vi "Interpolated Fluid Properties.vi"(0 "Xi":dbl[](array[numeric]), 5 "Yi":dbl[](array[numeric]), 12 "file path (dialog if empty)":path=path "C:/LabView/CO2 properties from 250 to 400 K and 8 to 15 MPa.txt", 13 "reload?":bool) -> (8 "Zi 1":dbl[](array[numeric]), 10 "Zi 2":dbl[](array[numeric]), 15 "Zi 3":dbl[](array[numeric]))   [LabVIEW 2020]
uses:
  f9a0f065-e32f-4a9d-9d50-07fda239758b.vi
  fc243c30-5152-400b-8647-591f757cc8b1.vi
  5e9bb687-0e7f-4660-b8cc-9489864c6cfa.vi
  <vilib>/Utility/file.llb/Read Delimited Spreadsheet (DBL).vi
  <vilib>/gmath/interp.llb/Interpolate 2D Scattered (1D).vi
  <vilib>/gmath/NI_AAL_Interpolation.lvlib
panel:
  out "Heartbeat":u32(knob) scale=0.0..1000.0 scale format="%#.0f"
  in  "stop":bool
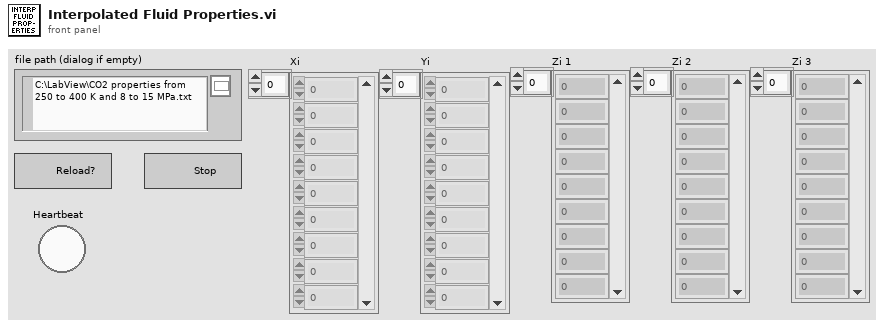
[diagram p1: front panel]
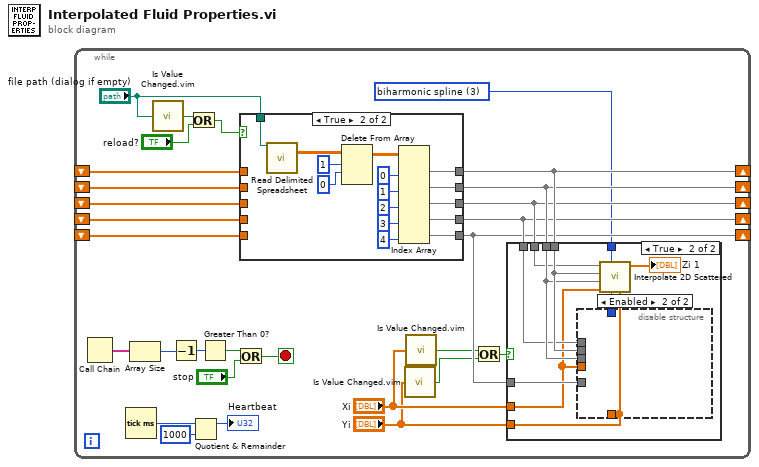
[diagram p0: block diagram]
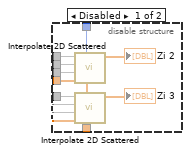
[diagram p3: hidden frame]
diagram:
  n1 = while {
    shift-right: [w25] -> _
    shift-left: _ -> [w20]
    shift-right: [w26] -> _
    shift-left: _ -> [w21]
    shift-right: [w27] -> _
    shift-left: _ -> [w22]
    shift-right: [w29] -> _
    shift-left: _ -> [w24]
    shift-right: [w28] -> _
    shift-left: _ -> [w23]
    stop <- w13 stop-if-true
    w19 = 3 items=["nearest", "linear", "cubic", "biharmonic spline "] ("method")
    n2 = Call Chain() -> (call chain=w14:string[])
    n3 = Tick Count (ms)() -> (millisecond timer value=w8:u32)
    n4 = Array Size(array=w14) -> (size(s)=w15:i32)
    n5 = call "Is Value Changed.vim"("value"="file path (dialog if empty)") -> ("changed or first call?"=w11:bool)
    n6 = Decrement(x=w15) -> (x-1=w16:i32)
    n7 = Or(x=w11, y="reload?") -> (x .or. y?=w10:bool)
    n8 = Quotient & Remainder(x=w8, y=u32 1000) -> (x-y*floor(x/y)=→"Heartbeat":u32)  [unwired: 1 out]
    n9 = Greater Than 0?(x=w16) -> (x > 0?=w17:bool)
    n10 = Or(x=w17, y="stop") -> (x .or. y?=w13:bool)
    n11 = case shown="True" w10 {
      tunnel: [w52 w61] -> w29
      tunnel: [w51 w60] -> w28
      tunnel: [w50 w59] -> w27
      tunnel: [w49 w58] -> w26
      tunnel: [w48 w57] -> w25
      tunnel: w24 -> [w52 _]
      tunnel: w23 -> [w51 _]
      tunnel: w22 -> [w50 _]
      tunnel: w21 -> [w49 _]
      tunnel: w20 -> [w48 _]
      tunnel: "file path (dialog if empty)" -> [_ w56]
      frame False {
      }
      frame True {
        n12 = call-poly <vilib>:"Read Delimited Spreadsheet.vi"("file path (dialog if empty)"=w56) -> ("all rows"=w67:dbl[][])  [unwired: 9 in, 5 out]
        n13 = Delete From Array(array=w67, length=1, index (row)=0) -> (array with subset deleted=w55:dbl[][])  [unwired: 1 in, 1 out]
        n14 = Index Array(array=w55, index (col) #1=0 ("disabled index (col)"), index (col) #2=1 ("index (col)"), index (col) #3=2 ("index (col)"), index (col) #4=3 ("index (col)"), index (col) #5=4 ("index (col)")) -> (element #1=w61:dbl[], element #2=w60:dbl[], element #3=w59:dbl[], element #4=w58:dbl[], element #5=w57:dbl[])  [unwired: 5 in]
      }
    }
    n15 = call "Is Value Changed.vim"("value"="Yi") -> ("changed or first call?"=w1:bool)
    n16 = call "Is Value Changed.vim"("value"="Xi") -> ("changed or first call?"=w2:bool)
    n17 = Or(x=w2, y=w1) -> (x .or. y?=w5:bool)
    n18 = case shown="True" w5 {
      tunnel: w29 -> [_ w38]
      tunnel: w28 -> [_ w37]
      tunnel: w27 -> [_ w36]
      tunnel: w26 -> [_ w35]
      tunnel: w25 -> [_ w34]
      tunnel: "Xi" -> [_ w33]
      tunnel: "Yi" -> [_ w32]
      tunnel: w19 -> [_ w31]
      frame False {
      }
      frame True {
        n19 = disable-structure shown="Enabled" {
          disable-tunnel: w38 -> [w47 _]
          disable-tunnel: w37 -> [w46 _]
          disable-tunnel: w35 -> [w45 _]
          disable-tunnel: w34 -> [w44 _]
          disable-tunnel: w33 -> [w43 _]
          disable-tunnel: w32 -> [w42 _]
          disable-tunnel: w31 -> [w41 _]
          frame Disabled {
            n20 = call-poly <vilib>:"Interpolate 2D Scattered.vi"("Yi"=w42, "method"=w41, "Xi"=w43, "Y"=w46, "X"=w47, "Z"=w45) -> ("Zi"=→"Zi 2":dbl[])  [unwired: 4 in, 1 out]
            n21 = call-poly <vilib>:"Interpolate 2D Scattered.vi"("Yi"=w42, "method"=w41, "Xi"=w43, "Y"=w46, "X"=w47, "Z"=w44) -> ("Zi"=→"Zi 3":dbl[])  [unwired: 4 in, 1 out]
          }
          frame Enabled {
          }
        }
        n22 = call-poly <vilib>:"Interpolate 2D Scattered.vi"("Yi"=w32, "method"=w31, "Xi"=w33, "Y"=w37, "X"=w38, "Z"=w36) -> ("Zi"=→"Zi 1":dbl[])  [unwired: 4 in, 1 out]
      }
    }
  }
